vi "Get Configurations.vi"(8 "error in (no error)":errorcluster, 11 "EPU452 in":refnum<class "EPU452.lvclass">) -> (0 "error out":errorcluster, 1 "Channel Configs":T1[](array[typedef]), 2 "Response":string, 3 "EPU452 out":refnum<class "EPU452.lvclass">)   [LabVIEW 2018, in "EPU452.lvclass"]
uses:
  EPU452.lvclass
  Controls/Channel Config.ctl
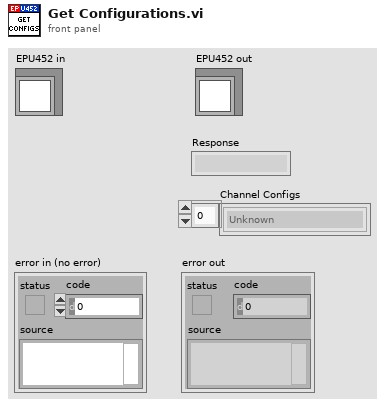
[diagram p1: front panel]
types:
  T1 = typedef "EPU452.lvclass/Channel Config.ctl" = enum16{"Unknown", "Disabled", "Voltmeter", "pH/ISE", "Pt 1k RTD", "10 k Thermistor", "dO2", "Biosensor", "Conductivity"}
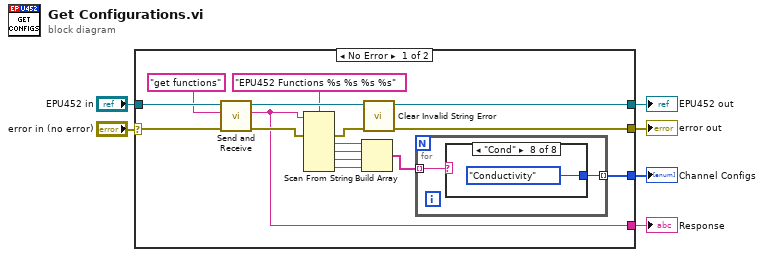
[diagram p0: block diagram]
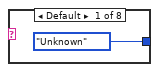
[diagram p2: hidden frame]
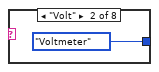
[diagram p3: hidden frame]
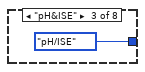
[diagram p4: hidden frame]
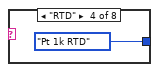
[diagram p5: hidden frame]
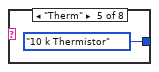
[diagram p6: hidden frame]
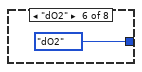
[diagram p7: hidden frame]
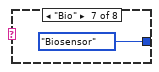
[diagram p8: hidden frame]
diagram:
  n1 = case shown="No Error" "error in (no error)" {
    selector: "error in (no error)" -> [w12 w34]
    tunnel: [w15 w34] -> w5
    tunnel: [w16 w33] -> w3
    tunnel: "EPU452 in" -> [w13 w33]
    tunnel: [w14 _] -> w2
    tunnel: [w7 _] -> w1
    frame No Error {
      n2 = call "Send and Receive.vi"("error in (no error)"=w12, "Command"="get functions" ("Function"), "EPU452 in"=w13) -> ("error out"=w8:errorcluster, "Response"=w7:string, "EPU452 out"=w11:refnum<class "EPU452.lvclass">)  [unwired: 6 in]
      n3 = Scan From String(format string="EPU452 Functions %s %s %s %s", input string=w7, error in=w8) -> (error out=w18:errorcluster, output 1=w22:string, output 2=w21:string, output 3=w20:string, output 4=w19:string)  [unwired: 5 in, 2 out]
      n4 = Build Array(w22, w21, w20, w19) -> (w17:string[])
      n5 = call "Clear Invalid String Error.vi"("error in (no error)"=w18, "EPU452 in"=w11) -> ("error out"=w15:errorcluster, "EPU452 out"=w16:refnum<class "EPU452.lvclass">)  [unwired: 8 in]
      n6 = for {
        tunnel: w17 -> [w24] mode=indexing
        tunnel: [w23] -> w14 mode=indexing
        n7 = case shown="\"Cond\"" w24 {
          tunnel: [Channel_Config."Unknown" ("Channel Config") Channel_Config."Voltmeter" ("Channel Config") Channel_Config."pH/ISE" ("Channel Config") Channel_Config."Pt 1k RTD" ("Channel Config") Channel_Config."10 k Thermistor" ("Channel Config") Channel_Config."dO2" ("Channel Config") Channel_Config."Biosensor" ("Channel Config") Channel_Config."Conductivity" ("Channel Config")] -> w23
          frame Default {
          }
          frame "Volt" {
          }
          frame "pH&ISE" {
          }
          frame "RTD" {
          }
          frame "Therm" {
          }
          frame "dO2" {
          }
          frame "Bio" {
          }
          frame "Cond" {
          }
        }
      }
    }
    frame Error {
    }
  }
  "error out" <- w5
  "EPU452 out" <- w3
  "Channel Configs" <- w2
  "Response" <- w1
